vi "DB Insert Query.vi"(6 "FP Data":string[](array[string]), 7 "TableName":string, 8 "error in (no error)":errorcluster, 9 "DB Column Name":string[](array[string]), 10 "Schema":string="edcu_ltt", 11 "Database in":refnum<class "MYSQL Server.lvclass">) -> (0 "error out":errorcluster, 2 "Query":string, 3 "Database out":refnum<class "MYSQL Server.lvclass">)   [LabVIEW 2023, in "HardwareAbstractionLayer_LVOOP.lvlib" / "MYSQL Server.lvclass"]
uses:
  MYSQL Server.lvclass
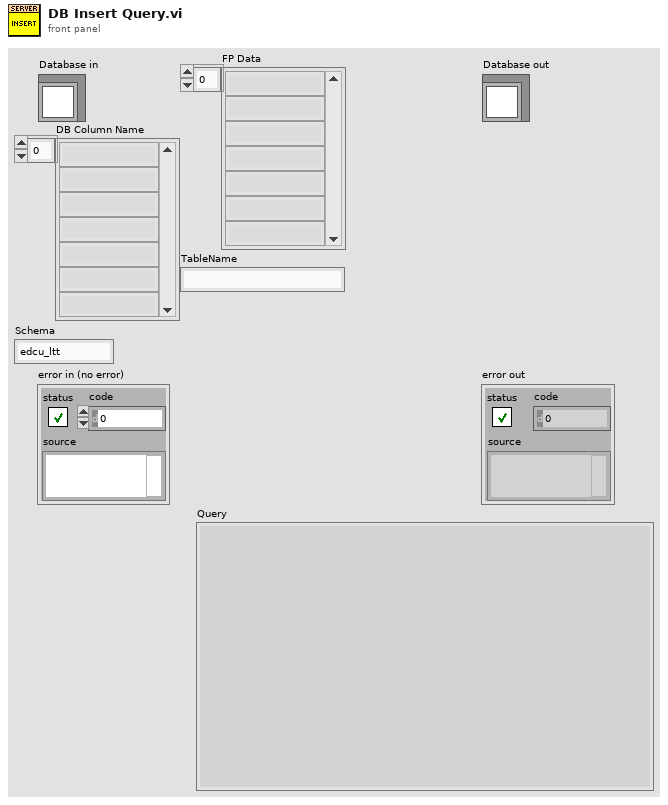
[diagram p1: front panel]
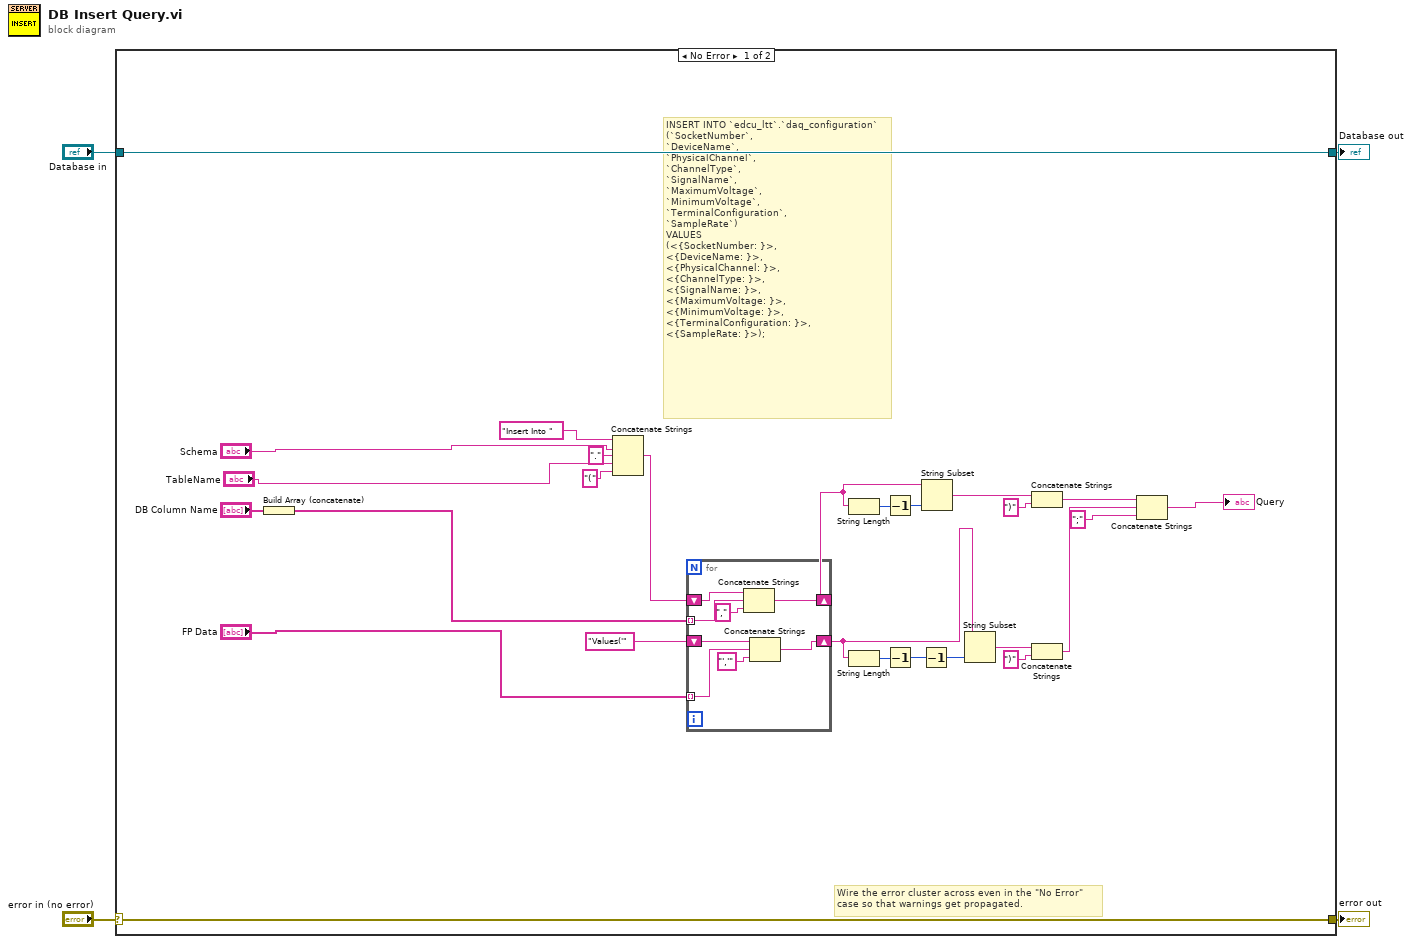
[diagram p0: block diagram]
diagram:
  n1 = case shown="No Error" "error in (no error)" {
    selector: "error in (no error)" -> [w30 w41]
    tunnel: [w30 w41] -> w3
    tunnel: [w31 w40] -> w1
    tunnel: "Database in" -> [w31 w40]
    frame No Error {
      # "INSERT INTO `edcu_ltt`.`daq_configuration`\n(`SocketNumber`,\n`DeviceName`,\n`PhysicalChannel`,\n`ChannelType`,\n`SignalName`,\n`MaximumVoltage`,\n`MinimumVoltage`,\n`TerminalConfiguration`,\n`SampleRate`)\nVALUES\n(<{SocketNumber: }>,\n<{DeviceName: }>,\n<{PhysicalChannel: }>,\n<{ChannelType: }>,\n<{SignalName: }>,\n<{MaximumVoltage: }>,\n<{MinimumVoltage: }>,\n<{TerminalConfiguration: }>,\n<{SampleRate: }>);"
      # "Wire the error cluster across even in the \"No Error\"\ncase so that warnings get propagated."
      n2 = Build Array (concatenate)("DB Column Name") -> (w26:string[])
      n3 = Concatenate Strings("Insert Into " ("string"), "Schema", "." ("string"), "TableName", "(" ("string")) -> (w22:string)
      n4 = for {
        shift-right: [w36] -> w18
        shift-left: w22 -> [w39]
        tunnel: w26 -> [w38] mode=indexing
        shift-right: [w32] -> w14
        shift-left: "Values('" -> [w35]
        tunnel: "FP Data" -> [w34] mode=indexing
        n5 = Concatenate Strings(w39, w38, "," ("string")) -> (w36:string)
        n6 = Concatenate Strings(w35, w34, "','" ("string")) -> (w32:string)
      }
      n7 = String Length(string=w18) -> (length=w20:i32)
      n8 = String Length(string=w14) -> (length=w17:i32)
      n9 = Decrement(x=w20) -> (x-1=w19:i32)
      n10 = Decrement(x=w17) -> (x-1=w16:i32)
      n11 = Decrement(x=w16) -> (x-1=w15:i32)
      n12 = String Subset(string=w18, length (rest)=w19) -> (substring=w13:string)  [unwired: 1 in]
      n13 = String Subset(string=w14, length (rest)=w15) -> (substring=w11:string)  [unwired: 1 in]
      n14 = Concatenate Strings(w13, ")" ("string")) -> (w9:string)
      n15 = Concatenate Strings(w11, ")" ("string")) -> (w8:string)
      n16 = Concatenate Strings(w9, w8, ";" ("string")) -> (→"Query":string)
    }
    frame Error {
    }
  }
  "error out" <- w3
  "Database out" <- w1
